vi "RIFORMATTA DATA.vi"(10 "time stamp":timestamp) -> (2 "DATA RIFORMATTATA":string)   [LabVIEW 2019]
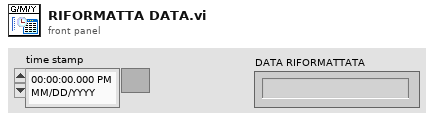
[diagram p1: front panel]
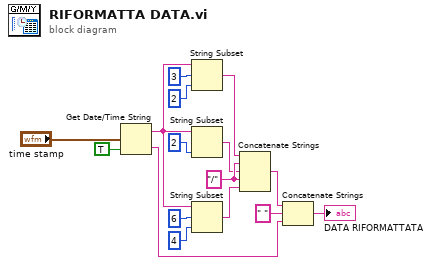
[diagram p0: block diagram]
diagram:
  w7 = "/" ("string")
  n1 = Get Date/Time String(seconds (now)="time stamp", want seconds? (F)=TRUE) -> (date string=w2:string, time string=w13:string)  [unwired: 1 in]
  n2 = String Subset(string=w2, offset (0)=3, length (rest)=2 ("length (rest)")) -> (substring=w5:string)
  n3 = String Subset(string=w2, length (rest)=2 ("length (rest)")) -> (substring=w6:string)  [unwired: 1 in]
  n4 = String Subset(string=w2, offset (0)=6, length (rest)=4 ("length (rest)")) -> (substring=w4:string)
  n5 = Concatenate Strings(w5, w7, w6, w7, w4) -> (w1:string)
  n6 = Concatenate Strings(w1, " " ("string"), w13) -> (→"DATA RIFORMATTATA":string)
